vi "Remove.vi"(8 "error in (no error)":errorcluster, 9 "Role":string, 10 "Action":string, 11 "Policies in":refnum<class "Policies.lvclass">) -> (0 "error out":errorcluster, 3 "Policies out":refnum<class "Policies.lvclass">)   [LabVIEW 2016, in "Policies.lvclass"]
uses:
  Policies.lvclass
  Policies.lvclass/Policies.ctl
  LUT/LUT.lvclass
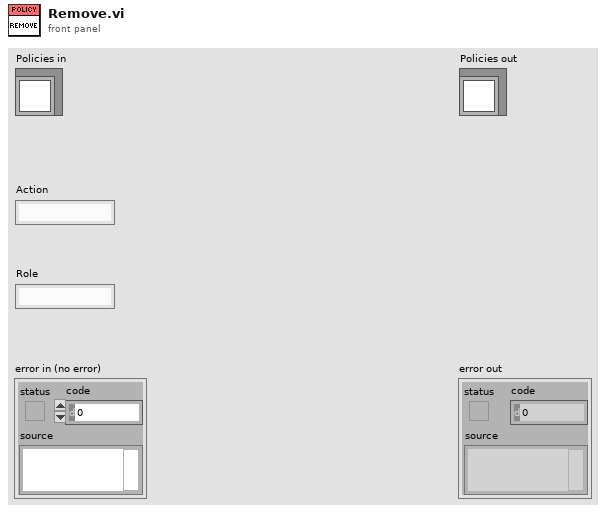
[diagram p1: front panel]
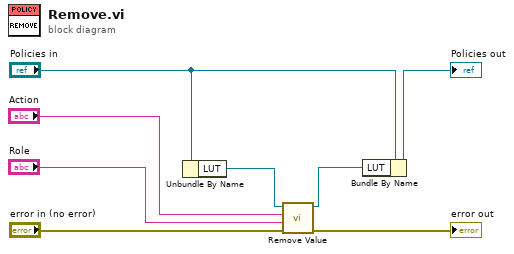
[diagram p0: block diagram]
diagram:
  n1 = Unbundle By Name("Policies in") -> ("LUT"=w6:refnum<class "LUT.lvclass">)
  n2 = call "Remove Value.vi"("error in (no error)"="error in (no error)", "Value"="Role", "Key"="Action", "LUT in"=w6) -> ("error out"=→"error out":errorcluster, "LUT out"=w5:refnum<class "LUT.lvclass">)  [unwired: 6 in]
  n3 = Bundle By Name(cluster="Policies in", "LUT"=w5) -> (→"Policies out":refnum<class "Policies.lvclass">)
